vi "stop.vi"(8 "error in (no error)":errorcluster, 10 "stop":bool, 11 "niDAQmxDO in":refnum<class "niDAQmxDO.lvclass">) -> (0 "error out":errorcluster, 2 "stopped":bool, 3 "niDAQmxDO out":refnum<class "niDAQmxDO.lvclass">)   [LabVIEW 2009, in "Hardware.lvlib" / "Channels.lvlib" / "niDAQmxDO.lvclass"]
uses:
  niDAQmxDO.lvclass
panel:
  out "for testing only":bool=TRUE
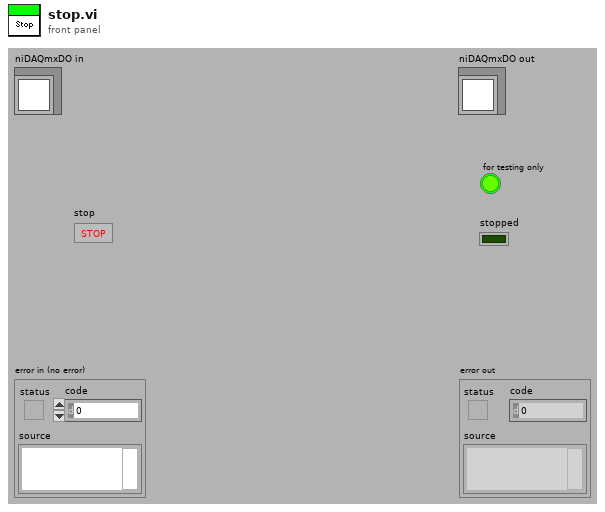
[diagram p1: front panel]
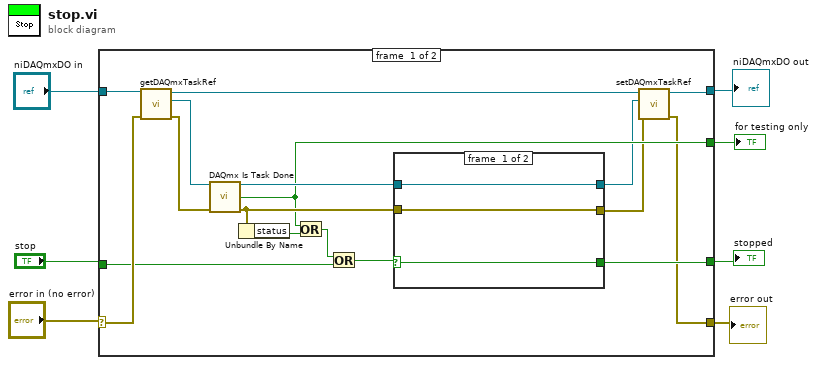
[diagram p0: block diagram]
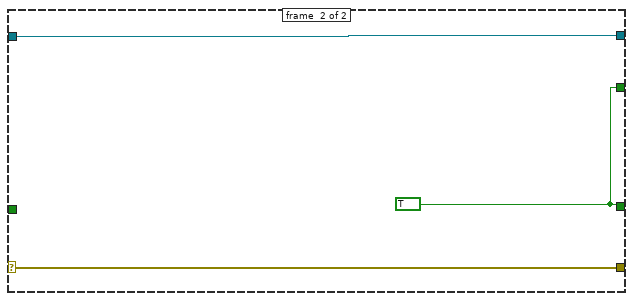
[diagram p3: hidden frame]
diagram:
  n1 = case shown="No Error" "error in (no error)" {
    selector: "error in (no error)" -> [w23 w32]
    tunnel: "niDAQmxDO in" -> [w24 w33]
    tunnel: [w12 w33] -> w5
    tunnel: [w8 w32] -> w4
    tunnel: "stop" -> [w15 _]
    tunnel: [w14 w31] -> w2
    tunnel: [w13 w31] -> w1
    frame #0 {
      n2 = call "getDAQmxTaskRef.vi"("error in (no error)"=w23, "niDAQmxDO.lvclass in"=w24) -> ("error out"=w16:errorcluster, "DAQmx Task Ref"=w17:refnum<k21>, "niDAQmxDO.lvclass out"=w11:refnum<class "niDAQmxDO.lvclass">)  [unwired: 7 in]
      n3 = call <vilib>:"DAQmx Is Task Done.vi"("task/channels in"=w17, "error in"=w16) -> ("task out"=w22:refnum<k21>, "task done?"=w14:bool, "error out"=w21:errorcluster)  [unwired: 11 in]
      n4 = Unbundle By Name(w21) -> ("status"=w19:bool)
      n5 = Or(x=w14, y=w19) -> (x .or. y?=w20:bool)
      n6 = Or(x=w20, y=w15) -> (x .or. y?=w18:bool)
      n7 = case shown="False" w18 {
        selector: w18 -> [w26 w30]
        tunnel: w22 -> [w25 w28]
        tunnel: w21 -> [w27 w29]
        tunnel: [w27 w29] -> w9
        tunnel: [w26 w30] -> w13
        tunnel: [w25 w28] -> w10
        frame #0 {
        }
        frame #1 {
        }
      }
      n8 = call "setDAQmxTaskRef.vi"("error in (no error)"=w9, "DAQmx Task Ref"=w10, "niDAQmxDO.lvclass in"=w11) -> ("error out"=w8:errorcluster, "niDAQmxDO.lvclass out"=w12:refnum<class "niDAQmxDO.lvclass">)  [unwired: 7 in]
    }
    frame #1 {
      w31 = TRUE
    }
  }
  "error out" <- w4
  "niDAQmxDO out" <- w5
  "stopped" <- w1
  "for testing only" <- w2
